vi "Update Graphs.vi"(8 "error in (no error)":errorcluster, 11 "Sensor & Control in":refnum<class "Sensor.lvclass">) -> (0 "error out":errorcluster, 3 "Sensor & Control out":refnum<class "Sensor.lvclass">)   [LabVIEW 2013, in "Sensor.lvib.lvlib" / "Sensor.lvclass"]
uses:
  Sensor.lvclass
  Sensor.lvclass/Sensor.ctl
  Read Graph History.vi
  Read Graph.vi
  PluginInterface/PluginInterface.lvlibp/PluginInterfaceClass/Read TDMS.vi
  PluginInterface/PluginInterface.lvlibp/PluginInterfaceClass/Read Name.vi
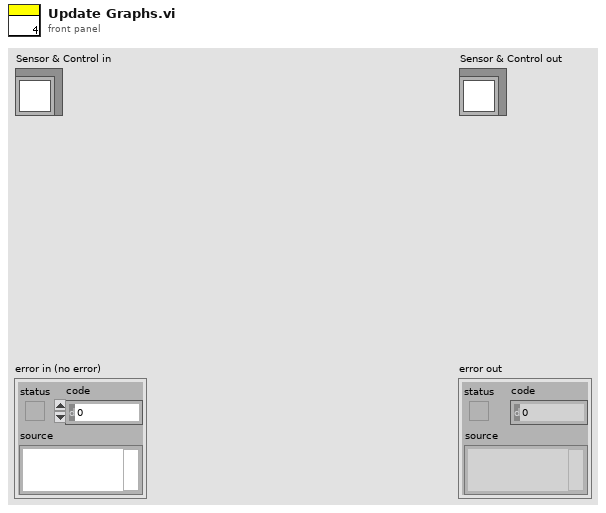
[diagram p1: front panel]
types:
  T1 = cluster{"output array":dbl[], "output array":dbl[]}
  T2 = cluster{"output array":dbl[], "output array":dbl[]}[]
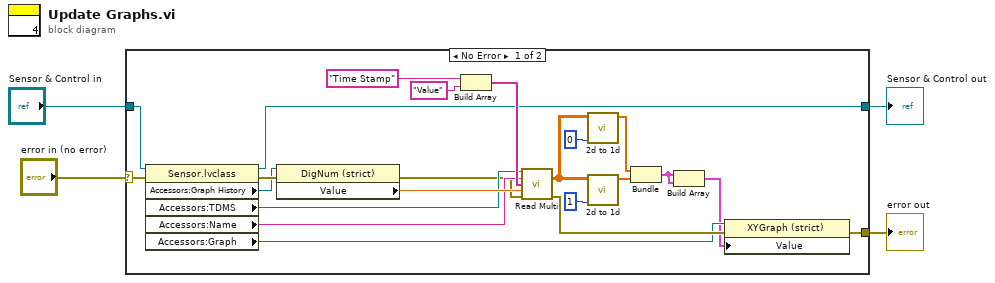
[diagram p0: block diagram]
diagram:
  n1 = case shown="No Error" "error in (no error)" {
    selector: "error in (no error)" -> [w23 w28]
    tunnel: [w10 w28] -> w1
    tunnel: [w7 w27] -> w2
    tunnel: "Sensor & Control in" -> [w26 w27]
    frame No Error {
      n2 = property class="Sensor.lvclass"(reference=w26, error in=w23) -> (reference out=w7:refnum<class "Sensor.lvclass">, error out=w22:errorcluster, "Accessors:Graph History"=w18:refnum<vi>, "Accessors:TDMS"=w19:refnum<k34>, "Accessors:Name"=w9:string, "Accessors:Graph"=w16:refnum<vi>)
      n3 = property class="DigNum (strict)"(reference=w18, error in=w22) -> (error out=w8:errorcluster, "Value"=w20:dbl)  [unwired: 1 out]
      n4 = Build Array("Time Stamp" ("Channel"), "Value" ("string")) -> (w21:string[])
      n5 = call "Read Multi.vi"("tdms file in"=w19, "group"=w9, "Channel"=w21, "Numeric"=w20, "error in (no error)"=w8) -> ("Array"=w5:dbl[][], "error out"=w17:errorcluster)  [unwired: 7 in, 2 out]
      n6 = call "2d to 1d.vi"("index"=0, "array"=w5) -> ("output array"=w13:dbl[])  [unwired: 9 in]
      n7 = call "2d to 1d.vi"("index"=1, "array"=w5) -> ("output array"=w11:dbl[])  [unwired: 9 in]
      n8 = Bundle("output array"=w13, "output array"=w11) -> (w6:T1)  [unwired: 1 in]
      n9 = Build Array(w6, w6) -> (w12:T2)
      n10 = property class="XYGraph (strict)"(reference=w16, error in=w17, "Value"=w12) -> (error out=w10:errorcluster)  [unwired: 1 out]
    }
    frame Error {
    }
  }
  "error out" <- w1
  "Sensor & Control out" <- w2
